vi "FindMinimumChiSquaredFast.vi"(2 "Restrict to Positive Imaginary Part":bool=TRUE, 3 "Starting points 2":dbl[][](array[numeric])=[[1.5, 0.1], [1.5, 0.11], [1.52, 0.1]], 4 "Simplex Graph":refnum<vi>, 5 "Extinction ExtinctionUncertainity Size parameter and Number ofS sizes":T1={"Extinction"=[1.9915476e-09, 2.5260327e-09, 2.9463496e-09, 3.6659398e-09, 4.1150909e-09, 4.3561701e-09, 4.8158371e-09, 5.5805258e-09], "Extinction Uncertainty"=[1.1685435e-10, 1.8562181e-10, 2.4682015e-10, 3.9807269e-10, 5.4913102e-10, 1.091901e-09, 1.2235488e-09, 1.7175431e-09], "Size parameters"=[2.4744035643168516, 2.699349342891111, 2.92429512146537, 3.149240900039629, 3.3741866786138885, 3.599132457188148, 3.8240782357624066, 4.049024014336666], "Number ofSizes"=8.0, "GeometricCrossSection"=[5.939573610693203e-10, 7.068583470577035e-10, 8.295768100885549e-10, 9.621127501618742e-10, 1.1044661672776617e-09, 1.2566370614359174e-09, 1.418625432636641e-09, 1.590431280879833e-09], "Wave Length"=349.14999, "SMPS Sizes"=[105.5, 109.4, 113.4, 117.6, 121.9, 126.3, 131.0, 135.8, 140.7, 145.9, 151.2, 156.8, 162.5, 168.5, 174.7, 181.1, 187.7, 194.6, 201.7, 209.1, 216.7, 224.7, 232.9, 241.4, 250.3, 259.5, 269.0, 278.8, 289.0, 299.6, 310.6, 322.0, 333.8, 346.0, 358.7, 371.8, 385.4, 399.5, 414.2, 429.4, 445.1, 461.4, 478.3, 495.8, 514.0, 532.8, 552.3, 572.5, 593.5, 615.3, 637.8, 661.2, 685.4, 710.5, 736.5, 763.5, 791.5], "Concentration"=array8x57[456 elements], "Double Charge Correction"=TRUE, "Extincation Factor"=1.0, "Diameter Factor"=1.0, "Diameter Offset"=0.0, "Extinction Factor Flag"=FALSE, "Diameter Factor Flag"=FALSE, "Diameter Offset Flag"=FALSE, "Sizes"=[275.0, 300.0, 325.0, 350.0, 375.0, 400.0, 425.0, 450.0], "ExtinctionOrAbsorptionOrScattering"=0, "Convergence Strength"=enum."Weak"} {"ExtinctionOrAbsorptionOrScattering" scale=0.0..2.0}) -> (0 "Imaginary Part from fit":dbl=0.051495699826118665, 1 "Real Part from fit":dbl=1.57799797397569)   [LabVIEW 2013]
uses:
  BaesDataTypeDefinition.ctl
  RTDownhillSimplex.llb/RTDownhillSimplexGlobals.vi
panel:
  out "Waveform Chart":i32(graph)=60
  out "Starting points 3":dbl[][](array[numeric])=[[1.6630594557043747, 0.246532961950036], [1.4605000230939145, 0.15705446819563057], [1.5705619064033547, 0.05175990620612842]]
  in  "Downhill-Simplex parameters 2":T2={"alpha"=1.0, "beta"=0.5, "gamma"=2.0, "Maximum"=FALSE}
  out "Stopping condition flag":bool=TRUE
  out "x-y":dbl[](array[numeric])=[0.000168992022227199, 0.00018933075538369454]
  in  "buzzer":bool
  in  "Continous":bool=TRUE
  in  "sleep-time":dbl
  out "Simplex":cluster{dbl[], dbl[]}[](graph)=[{[1.57799797397569, 1.5778289819534628, 1.5778839622345557, 1.57799797397569], [0.051495699826118665, 0.05130636907073497, 0.05144020076942982, 0.051495699826118665]}]
  out "ValueInput":dbl=0.9201608571739257 format="%#_8g"
  out "ValueOutput":dbl=0.920166987183041 format="%#_8g"
  out "newSimplexPoint":dbl[](array[numeric])=[1.57799797397569, 0.051495699826118665]
  in  "Testfunction":enum16{"Rosenbrock function", "PID Controller"}(ring)=enum."PID Controller"
  in  "Downhill-Simplex parameters":T2={"alpha"=1.0, "beta"=0.5, "gamma"=2.0, "Maximum"=FALSE}
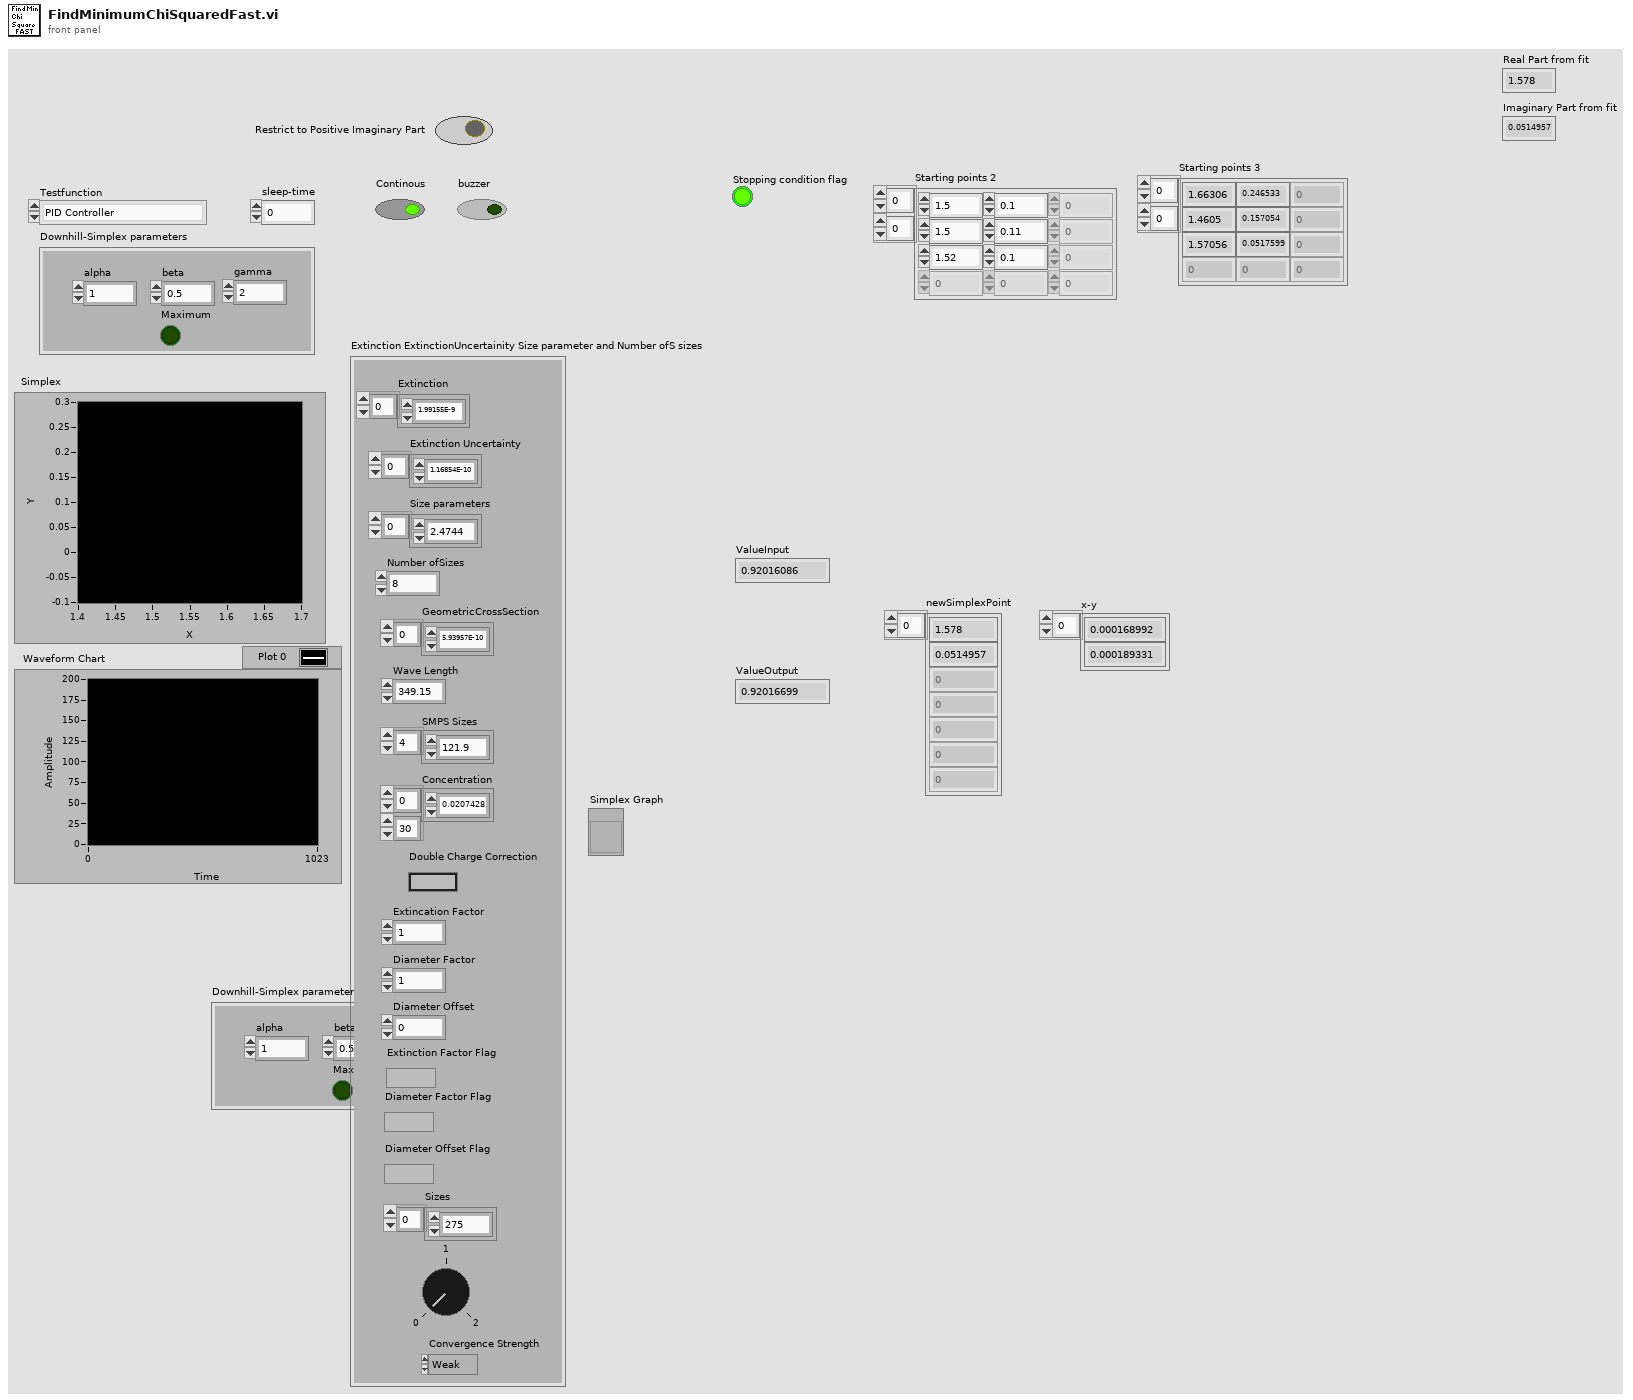
[diagram p1: front panel]
types:
  T1 = typedef "BaesDataTypeDefinition.ctl" = cluster{"Extinction":dbl[], "Extinction Uncertainty":dbl[], "Size parameters":dbl[], "Number ofSizes":dbl, "GeometricCrossSection":dbl[], "Wave Length":dbl, "SMPS Sizes":dbl[], "Concentration":dbl[][], "Double Charge Correction":bool, "Extincation Factor":dbl, "Diameter Factor":dbl, "Diameter Offset":dbl, "Extinction Factor Flag":bool, "Diameter Factor Flag":bool, "Diameter Offset Flag":bool, "Sizes":dbl[], "ExtinctionOrAbsorptionOrScattering":i8, "Convergence Strength":enum16{"Weak", "Medium", "Strong"}}
  T2 = cluster{"alpha":dbl, "beta":dbl, "gamma":dbl, "Maximum":bool}
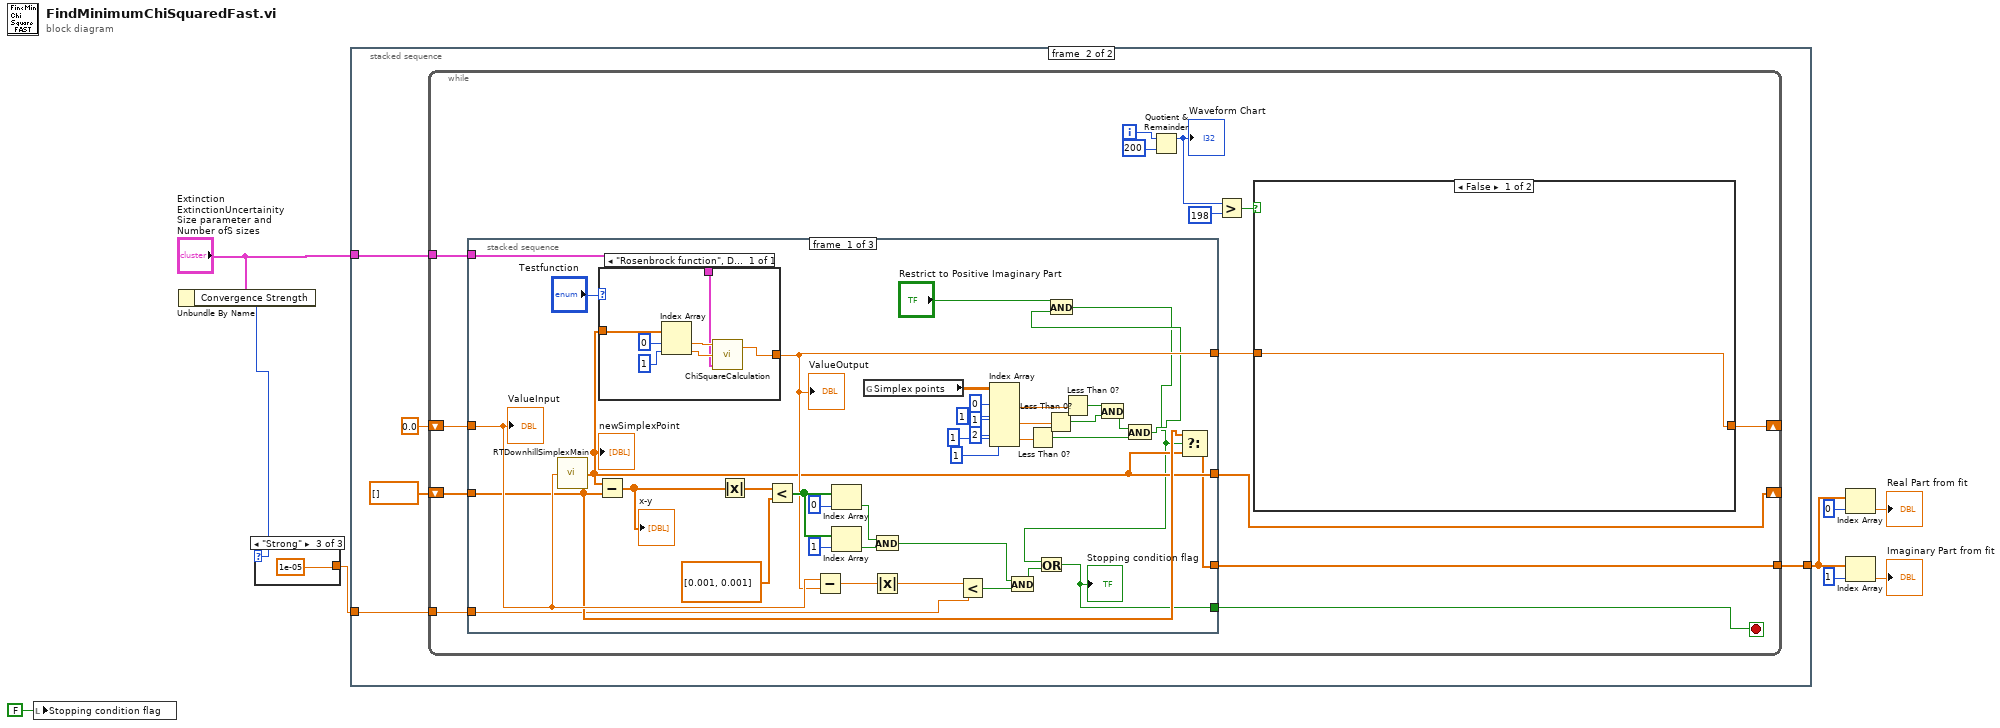
[diagram p0: block diagram]
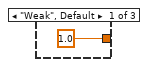
[diagram p2: hidden frame]
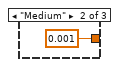
[diagram p3: hidden frame]
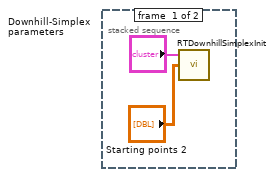
[diagram p4: hidden frame]
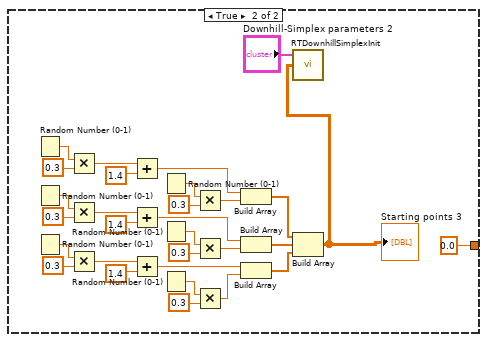
[diagram p5: hidden frame]
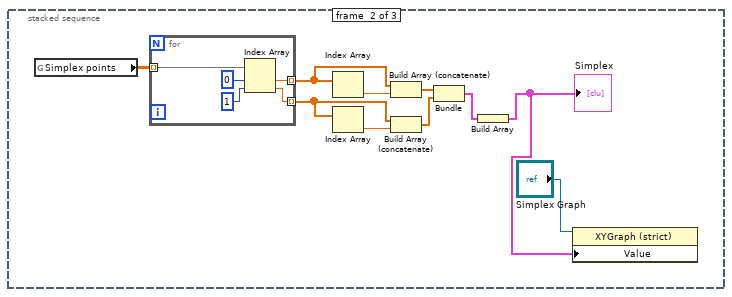
[diagram p6: hidden frame]
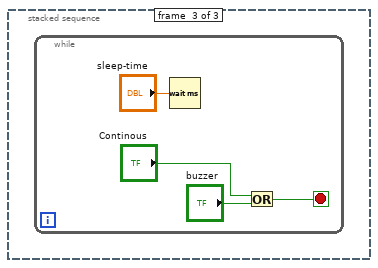
[diagram p7: hidden frame]
diagram:
  n1 = local write "Stopping condition flag"(FALSE ("Stopping condition flag")) -> ()
  n2 = Unbundle By Name("Extinction ExtinctionUncertainity Size parameter and Number ofS sizes") -> ("Convergence Strength"=w2:enum16{"Weak", "Medium", "Strong"})
  n3 = case shown="\"Strong\"" w2 {
    tunnel: [1.0 0.001 1e-05] -> w1
    frame "Weak", Default {
    }
    frame "Medium" {
    }
    frame "Strong" {
    }
  }
  n4 = stacked-sequence {
    tunnel: [_ w17] -> w6
    tunnel: "Extinction ExtinctionUncertainity Size parameter and Number ofS sizes" -> [_ w16]
    tunnel: w1 -> [_ w15]
    frame #0 {
      n5 = call "RTDownhillSimplexInit.vi"("Starting points"="Starting points 2", "Downhill-Simplex parameters"="Downhill-Simplex parameters") -> ()  [unwired: 2 in]
    }
    frame #1 {
      n6 = while {
        shift-right: [w26] -> _
        shift-left: 0.0 -> [w33]
        shift-right: [w32] -> _
        shift-left: dbl[] [] ("newSimplexPoint") -> [w31]
        tunnel: [w30] -> w17
        tunnel: w16 -> [w22]
        tunnel: w15 -> [w20]
        i -> [w25]
        stop <- w21 stop-if-true
        n7 = stacked-sequence {
          tunnel: w33 -> [w93 _ _]
          tunnel: [w92 _ _] -> w27
          tunnel: [w71 _ _] -> w32
          tunnel: w31 -> [w72 _ _]
          tunnel: [w70 _ _] -> w30
          tunnel: w22 -> [w88 _ _]
          tunnel: [w69 _ _] -> w21
          tunnel: w20 -> [w65 _ _]
          frame #0 {
            n8 = call "RTDownhillSimplexMain.vi"("newSimplexValue"=w93) -> ("newSimplexPoint"=w71:dbl[])
            "newSimplexPoint" <- w71
            n9 = Subtract(x=w71, y=w72) -> (x-y=w102:dbl[])
            "x-y" <- w102
            n10 = case shown="\"Rosenbrock function\", Default" "Testfunction" {
              tunnel: w71 -> [w110]
              tunnel: [w105] -> w92
              tunnel: w88 -> [w104]
              frame "Rosenbrock function", Default {
                n11 = Index Array(array=w110, index #1=0 ("index"), index #2=1 ("index")) -> (element #1=w107:dbl, element #2=w106:dbl)
                n12 = call "ChiSquareCalculation.vi"("Extinction ExtinctionUncertainity Size parameter and Number ofS sizes 2"=w104, "refractive index, imaginary"=w106, "refractive index, real"=w107) -> ("Chi Squared"=w105:dbl)  [unwired: 1 out]
              }
            }
            "ValueOutput" <- w92
            n13 = Absolute Value(x=w102) -> (abs(x)=w101:dbl[])
            n14 = Less?(x=w101, y=dbl[] [0.001, 0.001]) -> (x < y?=w97:bool[])
            n15 = Subtract(x=w93, y=w92) -> (x-y=w94:dbl)
            n16 = Index Array(array=w97, index=0) -> (element=w96:bool)
            n17 = Index Array(array=w97, index=1) -> (element=w95:bool)
            n18 = global read "RTDownhillSimplexGlobals.vi" "Simplex points"() -> (w86:dbl[][])
            n19 = And(x=w96, y=w95) -> (x .and. y?=w90:bool)
            n20 = Absolute Value(x=w94) -> (abs(x)=w91:dbl)
            n21 = Less?(x=w91, y=w65) -> (x < y?=w89:bool)
            n22 = Index Array(array=w86, index (row) #1=0 ("index (row)"), index (col) #1=1 ("disabled index (col)"), index (row) #2=1 ("index (row)"), index (col) #2=1 ("disabled index (col)"), index (row) #3=2 ("index (row)"), index (col) #3=1 ("disabled index (col)")) -> (element #1=w79:dbl, element #2=w78:dbl, element #3=w77:dbl)
            n23 = And(x=w90, y=w89) -> (x .and. y?=w87:bool)
            n24 = Less Than 0?(x=w77) -> (x < 0?=w73:bool)
            n25 = Less Than 0?(x=w78) -> (x < 0?=w75:bool)
            n26 = Less Than 0?(x=w79) -> (x < 0?=w76:bool)
            n27 = And(x=w76, y=w75) -> (x .and. y?=w74:bool)
            n28 = And(x=w74, y=w73) -> (x .and. y?=w67:bool)
            n29 = And(x="Restrict to Positive Imaginary Part", y=w67) -> (x .and. y?=w66:bool)
            n30 = Or(x=w66, y=w87) -> (x .or. y?=w69:bool)
            "Stopping condition flag" <- w69
            n31 = Select(t=w72, s=w66, f=w71) -> (s? t:f=w70:dbl[])
            "ValueInput" <- w93
          }
          frame #1 {
            n32 = global read "RTDownhillSimplexGlobals.vi" "Simplex points"() -> (w114:dbl[][])
            n33 = for {
              tunnel: w114 -> [w125] mode=indexing
              tunnel: [w122] -> w119 mode=indexing
              tunnel: [w121] -> w116 mode=indexing
              n34 = Index Array(array=w125, index #1=0 ("index"), index #2=1 ("index")) -> (element #1=w122:dbl, element #2=w121:dbl)
            }
            n35 = Index Array(array=w119) -> (element=w120:dbl)  [unwired: 1 in]
            n36 = Index Array(array=w116) -> (element=w117:dbl)  [unwired: 1 in]
            n37 = Build Array (concatenate)(w119, w120) -> (w118:dbl[])
            n38 = Build Array (concatenate)(w116, w117) -> (w115:dbl[])
            n39 = Bundle(w118, w115) -> (w113:cluster{dbl[], dbl[]})  [unwired: 1 out]
            n40 = Build Array(w113) -> (w111:cluster{dbl[], dbl[]}[])
            "Simplex" <- w111
            n41 = property class="XYGraph (strict)"(reference="Simplex Graph", "Value"=w111) -> ()  [unwired: 1 in, 2 out]
          }
          frame #2 {
            n42 = while {
              stop <- w128 stop-if-true
              n43 = Wait (ms)(milliseconds to wait="sleep-time") -> ()  [unwired: 1 out]
              n44 = Or(x="Continous", y="buzzer") -> (x .or. y?=w128:bool)
            }
          }
        }
        n45 = Quotient & Remainder(x=w25, y=200) -> (x-y*floor(x/y)=w23:i32)  [unwired: 1 out]
        "Waveform Chart" <- w23
        n46 = Greater?(x=w23, y=198) -> (0:w28:bool)
        n47 = case shown="False" w28 {
          tunnel: [w34 0.0 ("Chi Squared")] -> w26
          tunnel: w27 -> [w34 _]
          frame False {
          }
          frame True {
            n48 = Random Number (0-1)() -> (number: 0 to 1=w53:dbl)
            n49 = Random Number (0-1)() -> (number: 0 to 1=w49:dbl)
            n50 = Random Number (0-1)() -> (number: 0 to 1=w45:dbl)
            n51 = Multiply(x=w53, y=0.3) -> (x*y=w51:dbl)
            n52 = Multiply(x=w49, y=0.3) -> (x*y=w47:dbl)
            n53 = Multiply(x=w45, y=0.3) -> (x*y=w43:dbl)
            n54 = Add(x=w51, y=1.4) -> (x+y=w41:dbl)
            n55 = Add(x=w47, y=1.4) -> (x+y=w39:dbl)
            n56 = Add(x=w43, y=1.4) -> (x+y=w37:dbl)
            n57 = Random Number (0-1)() -> (number: 0 to 1=w59:dbl)
            n58 = Random Number (0-1)() -> (number: 0 to 1=w57:dbl)
            n59 = Random Number (0-1)() -> (number: 0 to 1=w55:dbl)
            n60 = Multiply(x=w59, y=0.3) -> (x*y=w40:dbl)
            n61 = Multiply(x=w57, y=0.3) -> (x*y=w38:dbl)
            n62 = Multiply(x=w55, y=0.3) -> (x*y=w36:dbl)
            n63 = Build Array(w41, w40) -> (w62:dbl[])
            n64 = Build Array(w39, w38) -> (w61:dbl[])
            n65 = Build Array(w37, w36) -> (w60:dbl[])
            n66 = Build Array(w62, w61, w60) -> (w35:dbl[][])
            "Starting points 3" <- w35
            n67 = call "RTDownhillSimplexInit.vi"("Starting points"=w35, "Downhill-Simplex parameters"="Downhill-Simplex parameters 2") -> ()  [unwired: 2 in]
          }
        }
      }
    }
  }
  n68 = Index Array(array=w6, index=0) -> (element=→"Real Part from fit":dbl)
  n69 = Index Array(array=w6, index=1) -> (element=→"Imaginary Part from fit":dbl)
